vi "Add VI to class library.vi"(8 "Error In":errorcluster, 9 "VI Ref":refnum<vi>, 10 "New method path":path, 11 "Class Ref":refnum<vi>) -> (0 "Error Out":errorcluster)   [LabVIEW 2013, in "Scripter.lvlib"]
uses:
  Scripter.lvlib
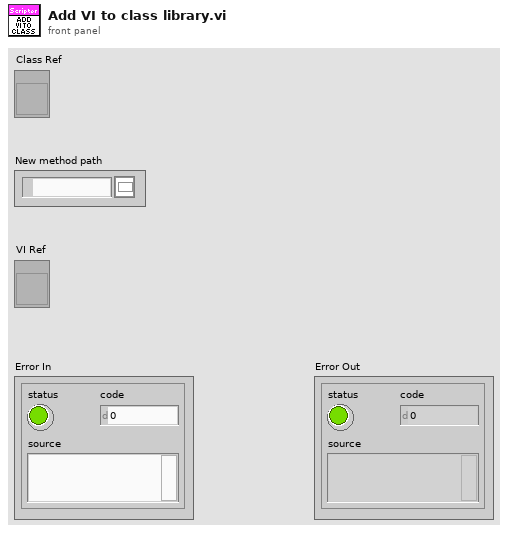
[diagram p1: front panel]
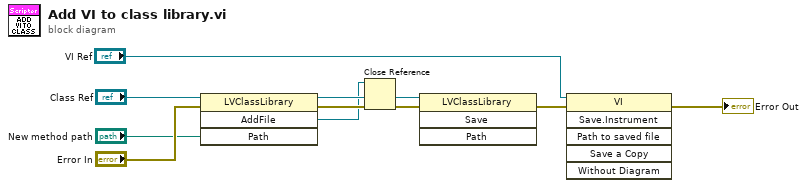
[diagram p0: block diagram]
diagram:
  n1 = invoke class="LVClassLibrary" method="AddFile"(reference="Class Ref", error in="Error In", "Path"="New method path") -> (reference out=w8:refnum<vi>, error out=w7:errorcluster, "AddFile"=w4:refnum<vi>)  [unwired: 1 in, 1 out]
  n2 = Close Reference(reference=w4, error in (no error)=w7) -> (error out=w5:errorcluster)
  n3 = invoke class="LVClassLibrary" method="Save"(reference=w8, error in=w5) -> (error out=w6:errorcluster)  [unwired: 2 in, 3 out]
  n4 = invoke class="VI" method="Save.Instrument"(reference="VI Ref", error in=w6) -> (error out=→"Error Out":errorcluster)  [unwired: 4 in, 5 out]
